vi "Disabled.vi"(7 "Robot Mode":T2, 10 "Match Info":T1={"Autonomous Elapsed Seconds"=0.0, "TeleOp Elapsed Seconds"=0.0, "Disabled Elapsed Seconds"=0.0, "Visited Autonomous"=FALSE, "Visited TeleOp"=FALSE, "Visited Disabled"=FALSE, "Autonomous Settings"={"Autonomous Style"=enum."Independent", "VI Refnum"=refnum}}, 11 "Call Context":T3) -> ()   [LabVIEW 2011]
doc: "This VI is called each time a disabled packet is received from the DS. It is often used to prepare for the next robot mode, to calibrate sensors, etc."
uses:
  <vilib>/Rock Robotics/WPI/DriverStation/WPI_DriverStationDerivedRobotMode.ctl
  <vilib>/Rock Robotics/WPI/DriverStation/WPI_DriverStationRobotMode.ctl
  <vilib>/Rock Robotics/WPI/DriverStation/WPI_DriverStationMatch Info.ctl
  Robot Global Data.vi
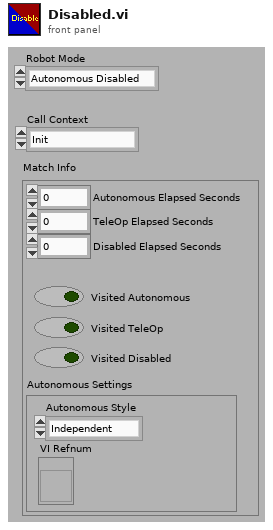
[diagram p1: front panel]
types:
  T1 = typedef "WPI_DriverStationMatch Info.ctl" = cluster{"Autonomous Elapsed Seconds":dbl, "TeleOp Elapsed Seconds":dbl, "Disabled Elapsed Seconds":dbl, "Visited Autonomous":bool, "Visited TeleOp":bool, "Visited Disabled":bool, "Autonomous Settings":cluster{"Autonomous Style":enum16{"Iterative", "Independent"}, "VI Refnum":refnum<vi>}}
  T2 = typedef "WPI_DriverStationRobotMode.ctl" = enum16{"Autonomous Disabled", "Autonomous Enabled", "Teleop Disabled", "Teleop Enabled", "Timeout", "Finish"}
  T3 = typedef "WPI_DriverStationDerivedRobotMode.ctl" = enum16{"Init", "Execute", "Stop"}
  T4 = typedef "WPI_JoystickDevRef.ctl" = cluster{"Device":T5}
  T5 = typedef "WPI_JoystickDeviceEnum.ctl" = enum16{"USB 1", "USB 2", "USB 3", "USB 4", "Kinect 1", "Kinect 2"}
  T6 = typedef "WPI_JoystickButtonState.ctl" = cluster{"Button 1":bool, "Button 2":bool, "Button 3":bool, "Button 4":bool, "Button 5":bool, "Button 6":bool, "Button 7":bool, "Button 8":bool, "Button 9":bool, "Button 10":bool, "Button 11":bool, "Button 12":bool}
  T7 = typedef "WPI_MotorControlDeviceRef.ctl" = cluster{"DeviceStatus":errorcluster, "Type":enum16{"PWM", "CAN"}, "PWM":cluster{"Digital Module":T8, "PWM Channel":T9, "DeadBand":T10}, "CAN":cluster{"Device Number":u8, "Control Mode":T11, "Semaphore":T12, "Max Vout":dbl}, "Invert":bool, "TransformRef":T13, "InvTransformRef":T13}
  T8 = typedef "FPGA_TypedefDigitalModule.ctl" = enum16{"Digital Module 1", "Digital Module 2"}
  T9 = typedef "FPGA_DIOPWMChannel.ctl" = enum8{"PWM 1", "PWM 2", "PWM 3", "PWM 4", "PWM 5", "PWM 6", "PWM 7", "PWM 8", "PWM 9", "PWM 10", "Invalid"}
  T10 = typedef "WPI_PWMDeadband.ctl" = cluster{"Name":string, "maxPositivePwm":i32, "minPositivePwm":i32, "centerPwm":i32, "maxNegativePwm":i32, "minNegativePwm":i32, "angularRange":u16}
  T11 = typedef "WPI_CANJaguar_ControlMode.ctl" = enum8{"Percent VBus", "Current", "Speed", "Position", "Voltage"}
  T12 = typedef "Semaphore RefNum" = refnum<k1>
  T13 = typedef "WPI_PWMTransform_ConPane.ctl" = refnum<vi>
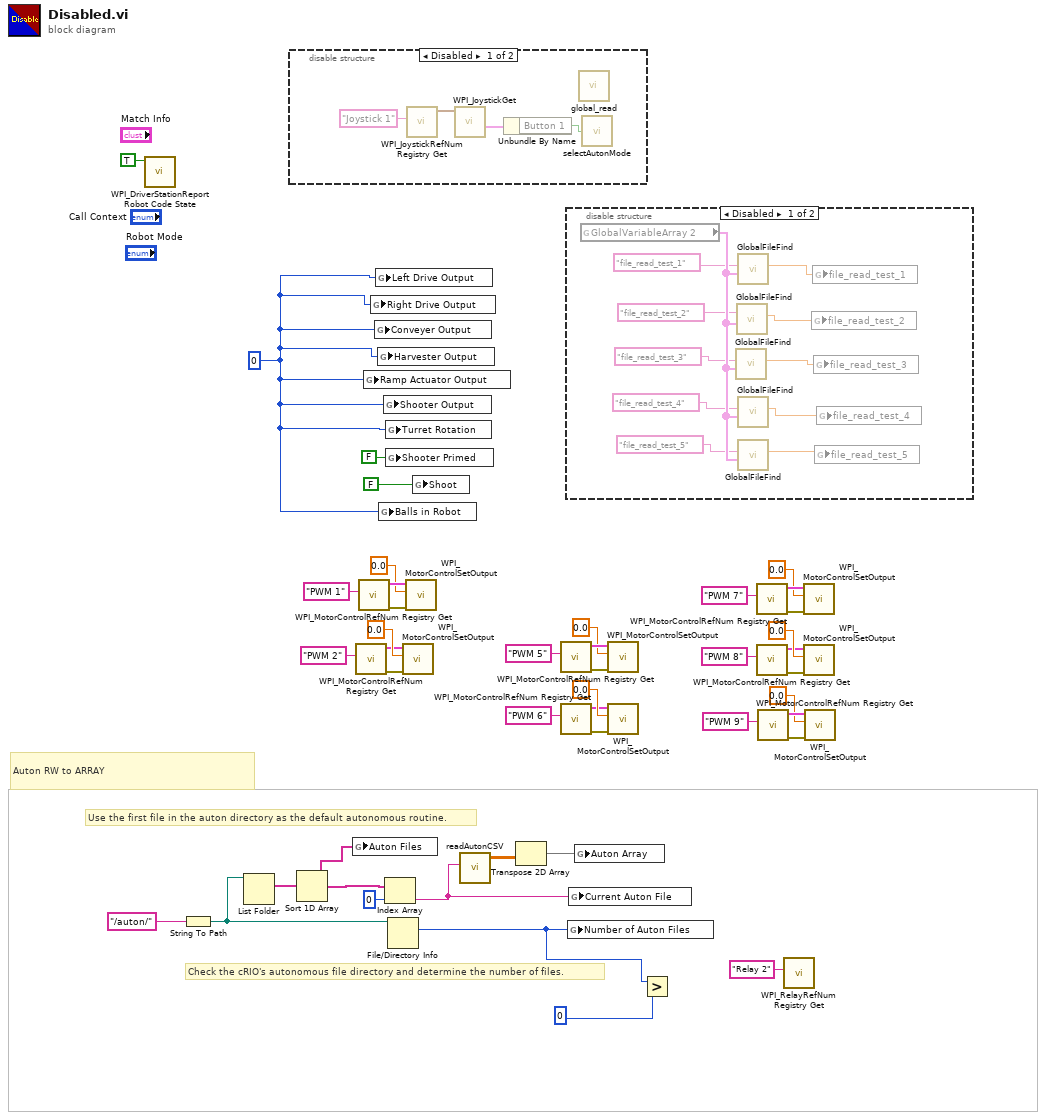
[diagram p0: block diagram]
diagram:
  w12 = 0
  # "Auton RW to ARRAY"
  # "Check the cRIO's autonomous file directory and determine the number of files."
  # "Use the first file in the auton directory as the default autonomous routine."
  n1 = call <vilib>:"WPI_DriverStationReport Robot Code State.vi"("Disabled"=TRUE ("Autonomous")) -> ()  [unwired: 10 in, 1 out]
  n2 = String To Path(string="/auton/") -> (path=w10:path)
  n3 = List Folder(path=w10) -> (filenames=w9:string[])  [unwired: 1 in, 5 out]
  n4 = disable-structure shown="Disabled" {
    frame Disabled {
      n5 = call <vilib>:"WPI_JoystickRefNum Registry Get.vi"("refnum name"="Joystick 1") -> ("JoystickDevRef"=w46:T4)  [unwired: 9 in, 1 out]
      n6 = call <vilib>:"WPI_JoystickGet.vi"("JoystickDevRef"=w46) -> ("Buttons"=w45:T6)  [unwired: 4 in, 2 out]
      n7 = Unbundle By Name(w45) -> ("Button 1"=w44:bool)
      n8 = call "global_read.vi"() -> ()  [unwired: 12 in]
      n9 = call "selectAutonMode.vi"("Joystick"=w44) -> ()  [unwired: 1 in]
    }
    frame Enabled {
    }
  }
  n10 = Sort 1D Array(array=w9) -> (sorted array=w7:string[])
  n11 = global write "Robot Global Data.vi" "Auton Files"(w7) -> ()
  n12 = call <vilib>:"WPI_MotorControlRefNum Registry Get.vi"("refnum name"="PWM 2") -> ("error out"=w36:errorcluster, "MotorControlDevRef"=w35:T7)  [unwired: 9 in]
  n13 = call <vilib>:"WPI_MotorControlRefNum Registry Get.vi"("refnum name"="PWM 1") -> ("error out"=w41:errorcluster, "MotorControlDevRef"=w42:T7)  [unwired: 9 in]
  n14 = global write "Robot Global Data.vi" "Ramp Actuator Output"(w12) -> ()
  n15 = global write "Robot Global Data.vi" "Right Drive Output"(w12) -> ()
  n16 = global write "Robot Global Data.vi" "Conveyer Output"(w12) -> ()
  n17 = global write "Robot Global Data.vi" "Left Drive Output"(w12) -> ()
  n18 = global write "Robot Global Data.vi" "Harvester Output"(w12) -> ()
  n19 = global write "Robot Global Data.vi" "Balls in Robot"(w12) -> ()
  n20 = global write "Robot Global Data.vi" "Shooter Output"(w12) -> ()
  n21 = Index Array(array=w7, index=0) -> (element=w4:string)
  n22 = global write "Robot Global Data.vi" "Turret Rotation"(w12) -> ()
  n23 = global write "Robot Global Data.vi" "Shooter Primed"(FALSE ("Shooter Primed")) -> ()
  n24 = File/Directory Info(path=w10) -> (size=w3:i64)  [unwired: 1 in, 6 out]
  n25 = call <vilib>:"WPI_MotorControlSetOutput.vi"("error in (no error)"=w36, "Output"=0.0, "MotorControlDevRef"=w35) -> ()  [unwired: 7 in, 2 out]
  n26 = call <vilib>:"WPI_MotorControlSetOutput.vi"("error in (no error)"=w41, "Output"=0.0, "MotorControlDevRef"=w42) -> ()  [unwired: 7 in, 2 out]
  n27 = global write "Robot Global Data.vi" "Shoot"(FALSE ("Shooter Primed")) -> ()
  n28 = call "readAutonCSV.vi"("AutonFile"=w4) -> ("AutonArray"=w6:dbl[][])  [unwired: 7 in]
  n29 = Transpose 2D Array(2D array=w6) -> (transposed array=w5:dbl[][])
  n30 = call <vilib>:"WPI_MotorControlRefNum Registry Get.vi"("refnum name"="PWM 5") -> ("error out"=w33:errorcluster, "MotorControlDevRef"=w34:T7)  [unwired: 9 in]
  n31 = call <vilib>:"WPI_MotorControlRefNum Registry Get.vi"("refnum name"="PWM 6") -> ("error out"=w28:errorcluster, "MotorControlDevRef"=w27:T7)  [unwired: 9 in]
  n32 = disable-structure shown="Disabled" {
    frame Disabled {
      n33 = global read "Robot Global Data.vi" "GlobalVariableArray 2"() -> (w58:cluster{"name":string, "va;":dbl}[])
      n34 = call "GlobalFileFind.vi"("GlobalVariableArray 2"=w58, "VariableNameLookup"="file_read_test_3") -> ("VariableValueOut"=w49:dbl)  [unwired: 9 in]
      n35 = call "GlobalFileFind.vi"("GlobalVariableArray 2"=w58, "VariableNameLookup"="file_read_test_2") -> ("VariableValueOut"=w48:dbl)  [unwired: 9 in]
      n36 = call "GlobalFileFind.vi"("GlobalVariableArray 2"=w58, "VariableNameLookup"="file_read_test_1") -> ("VariableValueOut"=w52:dbl)  [unwired: 9 in]
      n37 = call "GlobalFileFind.vi"("GlobalVariableArray 2"=w58, "VariableNameLookup"="file_read_test_4") -> ("VariableValueOut"=w50:dbl)  [unwired: 9 in]
      n38 = call "GlobalFileFind.vi"("GlobalVariableArray 2"=w58, "VariableNameLookup"="file_read_test_5") -> ("VariableValueOut"=w51:dbl)  [unwired: 9 in]
      n39 = global write "Robot Global Data.vi" "file_read_test_2"(w48) -> ()
      n40 = global write "Robot Global Data.vi" "file_read_test_1"(w52) -> ()
      n41 = global write "Robot Global Data.vi" "file_read_test_3"(w49) -> ()
      n42 = global write "Robot Global Data.vi" "file_read_test_5"(w51) -> ()
      n43 = global write "Robot Global Data.vi" "file_read_test_4"(w50) -> ()
    }
    frame Enabled {
    }
  }
  n44 = global write "Robot Global Data.vi" "Number of Auton Files"(w3) -> ()
  n45 = global write "Robot Global Data.vi" "Current Auton File"(w4) -> ()
  n46 = global write "Robot Global Data.vi" "Auton Array"(w5) -> ()
  n47 = call <vilib>:"WPI_MotorControlSetOutput.vi"("error in (no error)"=w33, "Output"=0.0, "MotorControlDevRef"=w34) -> ()  [unwired: 7 in, 2 out]
  n48 = call <vilib>:"WPI_MotorControlSetOutput.vi"("error in (no error)"=w28, "Output"=0.0, "MotorControlDevRef"=w27) -> ()  [unwired: 7 in, 2 out]
  n49 = Greater?(x=w3, y=i64 0) -> ()  [unwired: 1 out]
  n50 = call <vilib>:"WPI_MotorControlRefNum Registry Get.vi"("refnum name"="PWM 7") -> ("error out"=w25:errorcluster, "MotorControlDevRef"=w26:T7)  [unwired: 9 in]
  n51 = call <vilib>:"WPI_MotorControlRefNum Registry Get.vi"("refnum name"="PWM 8") -> ("error out"=w20:errorcluster, "MotorControlDevRef"=w19:T7)  [unwired: 9 in]
  n52 = call <vilib>:"WPI_MotorControlRefNum Registry Get.vi"("refnum name"="PWM 9") -> ("error out"=w17:errorcluster, "MotorControlDevRef"=w18:T7)  [unwired: 9 in]
  n53 = call <vilib>:"WPI_RelayRefNum Registry Get.vi"("refnum name"="Relay 2") -> ()  [unwired: 9 in, 2 out]
  n54 = call <vilib>:"WPI_MotorControlSetOutput.vi"("error in (no error)"=w25, "Output"=0.0, "MotorControlDevRef"=w26) -> ()  [unwired: 7 in, 2 out]
  n55 = call <vilib>:"WPI_MotorControlSetOutput.vi"("error in (no error)"=w20, "Output"=0.0, "MotorControlDevRef"=w19) -> ()  [unwired: 7 in, 2 out]
  n56 = call <vilib>:"WPI_MotorControlSetOutput.vi"("error in (no error)"=w17, "Output"=0.0, "MotorControlDevRef"=w18) -> ()  [unwired: 7 in, 2 out]
